vi "Unscale and Scale - Boolean.vi"(8 "error in (no error)":errorcluster, 11 "Data Scaling in":refnum<class "Data Scaling.lvclass">) -> (0 "error out":errorcluster, 3 "Data Scaling out":refnum<class "Data Scaling.lvclass">)   [LabVIEW 2020, in "Unit Tests.lvlib" / "Data Scaling.lvclass"]
uses:
  Data Scaling.lvclass
  Frames & Messages/TypeDefs/Scaling Information.ctl
  <vilib>/addons/_JKI Toolkits/Caraya/classes/Test/Test.lvclass
  <vilib>/addons/_JKI Toolkits/Caraya/classes/Assert/Assert.lvclass
  BCI-1553 API.lvlib
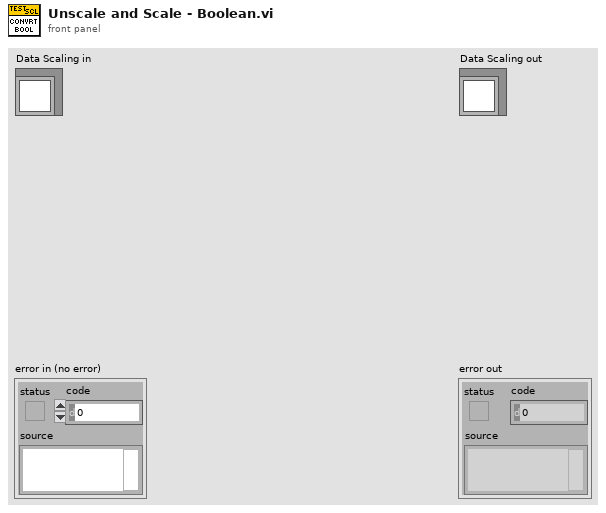
[diagram p1: front panel]
types:
  T1 = typedef "BCI-1553 API.lvlib/Scaling Information.ctl" = cluster{"Bit Offset":i32, "Bit Count":i32, "LSB Resolution":dbl, "2's Complement":bool, "Big Endian":bool, "Sign Bit":bool}
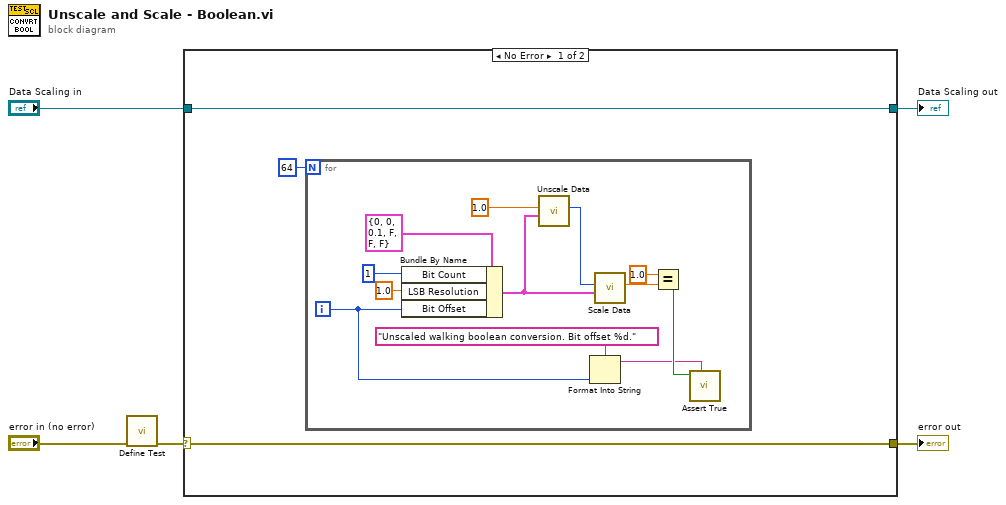
[diagram p0: block diagram]
diagram:
  n1 = call <vilib>:"Define Test.vi"("error in (no error)"="error in (no error)") -> ("error out"=w1:errorcluster)  [unwired: 9 in, 1 out]
  n2 = case shown="No Error" w1 {
    selector: w1 -> [w7 w22]
    tunnel: [w7 w22] -> w5
    tunnel: [w8 w21] -> w3
    tunnel: "Data Scaling in" -> [w8 w21]
    frame No Error {
      n3 = for {
        N: 64 -> [_]
        i -> [w9]
        n4 = Bundle By Name(cluster=T1 {"Bit Offset"=0, "Bit Count"=0, "LSB Resolution"=0.1, "2's Complement"=FALSE, "Big Endian"=FALSE, "Sign Bit"=FALSE} ("Scaling Info"), "Bit Count"=1, "LSB Resolution"=1.0, "Bit Offset"=w9) -> (w15:T1)
        n5 = call "Unscale Data.vi"("Scaling Info"=w15, "Scaled Value"=1.0 ("LSB Resolution")) -> ("Raw Value"=w17:u64)  [unwired: 8 in, 1 out]
        n6 = Format Into String(format string="Unscaled walking boolean conversion. Bit offset %d." ("Label"), w9) -> (resulting string=w10:string)  [unwired: 2 in, 1 out]
        n7 = call "Scale Data.vi"("Scaling Info"=w15, "Raw Value"=w17) -> ("Scaled Value"=w14:dbl)  [unwired: 8 in, 1 out]
        n8 = Equal?(x=1.0, y=w14) -> (x = y?=w12:bool)
        n9 = call <vilib>:"Assert True.vi"("Label"=w10, "True?"=w12) -> ()  [unwired: 8 in, 2 out]
      }
    }
    frame Error {
    }
  }
  "error out" <- w5
  "Data Scaling out" <- w3
